vi "NACA_0015_Post_Proc.vi"(3 "Mode":T5, 5 "Traverse line In":T2 {"Row Duration (mins)" format="%#.1f"; "Row No" min=0; "Trace Gas Concentration (%)" min=0.0 format="%#.2f"; "Emission Rate (l/min)" format="%#.2f"; "Tunnel Speed" format="%#.2f"; "Start X" format="%#.2f"; "Start Y" format="%#.2f"; "Start Z" format="%#.2f"; "End X" format="%#.2f"; "End Y" format="%#.2f"; "End Z" format="%#.2f"; "Averaging time (min)" min=0.0 format="%#.2f"}) -> (0 "Error Message":string, 1 "Status":T1, 2 "Traverse line Out":T2 {"Row Duration (mins)" format="%#.1f"; "Row No" min=0; "Trace Gas Concentration (%)" min=0.0 format="%#.2f"; "Emission Rate (l/min)" format="%#.2f"; "Tunnel Speed" format="%#.2f"; "Start X" format="%#.2f"; "Start Y" format="%#.2f"; "Start Z" format="%#.2f"; "End X" format="%#.2f"; "End Y" format="%#.2f"; "End Z" format="%#.2f"; "Averaging time (min)" min=0.0 format="%#.2f"})   [LabVIEW 2011]
uses:
  Gen Trav/Traverse_cluster.ctl
  Gen Trav/Spacing.ctl
  Controls/Multi_run_mode.ctl
  Controls/User_Specific_mode.ctl
  Gen Trav/Multi_Run_Status.ctl
  Controls/File_Selector_Type.ctl
  <vilib>/Analysis/8numeric.llb/1D Numeric Integration.vi
  <vilib>/Analysis/NI_AALPro.lvlib
panel:
  out "Array":dbl[][](array[numeric])
  # "X           Y            Z"
  # "Start"
  # "End"
  # "X           Y            Z"
  # "Start"
  # "End"
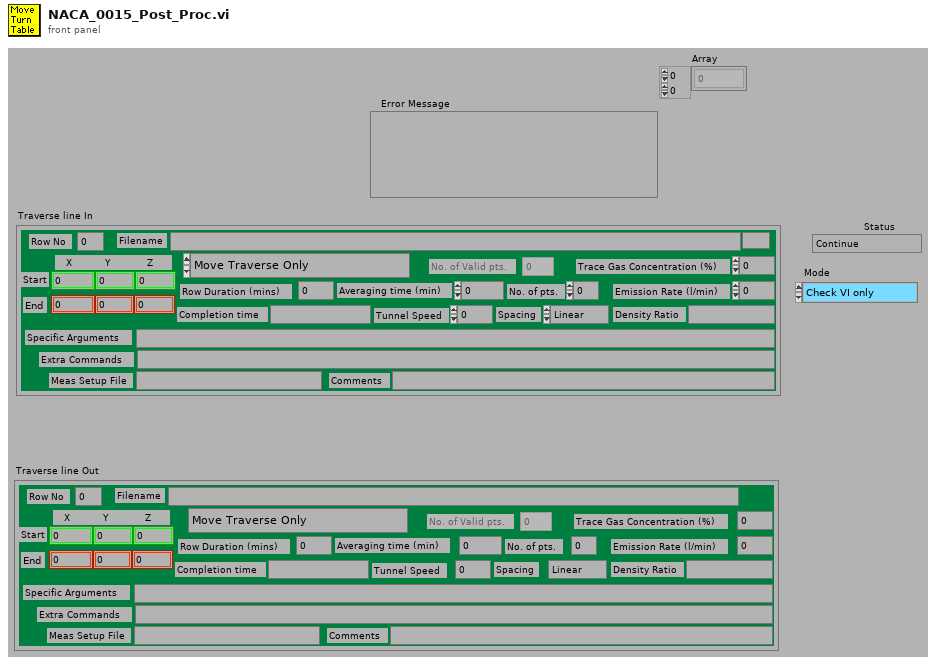
[diagram p1: front panel]
types:
  T1 = typedef "Multi_Run_Status.ctl" = enum16{"Continue", "Jump to Next Point", "Jump to Next Row", "Jump To Fall Back", "Terminate Run"}
  T2 = typedef "Traverse_cluster.ctl" = cluster{"Start X":dbl, "Start Y":dbl, "Start Z":dbl, "End X":dbl, "End Y":dbl, "End Z":dbl, "No. of pts.":i32, "Spacing":T3, "Filename":path, "Tunnel Speed":dbl, "Averaging time (min)":dbl, "Extra Commands":string, "Specific Arguments":string, "Emission Rate (l/min)":dbl, "Trace Gas Concentration (%)":dbl, "Density Ratio":string, "Comments":string, "Row No":i32, "Row Type Selector":T4, "Completion time":string, "Row Duration (mins)":dbl, "No. of Valid pts.":i32, "Meas Setup File":string}
  T3 = typedef "Spacing.ctl" = enum16{"Linear", "Log", "Gauss", "Specified", "N/A"}
  T4 = typedef "Multi_run_mode.ctl" = enum16{"Move Traverse Only", "Set Tunnel Speed Only", "Set Source Only", "Set Measurement Conditions", "Single Measurement", "Vertical Profile", "Lateral Profile", "Longitudinal Profile", "Explore Volume", "Multi-Axis Profile", "Auto Calibrate", "Meas Fast FID Bkgnd", "Check Beam Power", "Scanning Valve Measurement", "Run VI Named:", "Set ADAM Ch", "Wait (minutes)", "Send Message", "Synchronize With:", "Fall Back to this Row", "Turn Off Row Repeating", "Blank Row"}
  T5 = typedef "User_Specific_mode.ctl" = enum16{"Check VI only", "Run VI"}
  T6 = typedef "File_Selector_Type.ctl" = enum16{"The Selected File", "The Selected Folder", "Files containing the search string in the selected folder", "All files listed in selected file"}
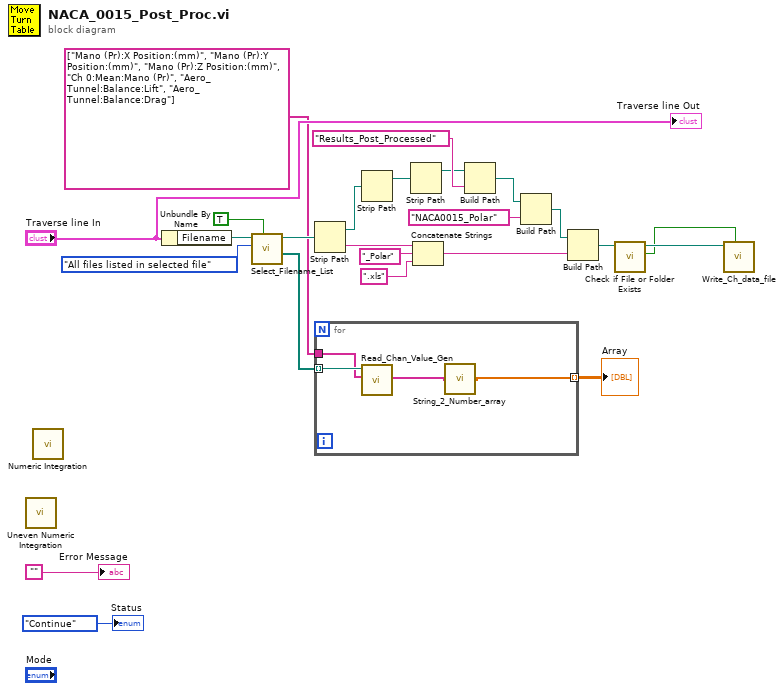
[diagram p0: block diagram]
diagram:
  n1 = call <vilib>:"Uneven Numeric Integration.vi"() -> ()  [unwired: 10 in, 2 out]
  n2 = call-poly <vilib>:"Numeric Integration.vi"() -> ()  [unwired: 3 in, 2 out]
  n3 = Unbundle By Name("Traverse line In") -> ("Filename"=w21:path)
  n4 = call "Select_Filename_List.vi"("No dialogs"=TRUE, "At Dialog Prompt Post Process"=File_Selector_Type."All files listed in selected file", "Previous Choice"=w21) -> ("Selected files"=w18:path[], "Choosen path"=w8:path)  [unwired: 3 in, 1 out]
  n5 = Strip Path(path=w8) -> (stripped path=w7:path, name=w6:string)
  n6 = for {
    tunnel: w18 -> [w28] mode=indexing
    tunnel: string[] ["Mano (Pr):X Position:(mm)", "Mano (Pr):Y Position:(mm)", "Mano (Pr):Z Position:(mm)", "Ch 0:Mean:Mano (Pr)", "Aero_Tunnel:Balance:Lift", "Aero_Tunnel:Balance:Drag"] -> [w27]
    tunnel: [w25] -> w1 mode=indexing
    n7 = call "Read_Chan_Value_Gen.vi"("Desired Ch Names"=w27, "Raw data file"=w28) -> ("Values"=w26:string[])  [unwired: 9 in]
    n8 = call "String_2_Number_array.vi"("Input String"=w26) -> ("Values"=w25:dbl[])
  }
  "Array" <- w1
  n9 = Strip Path(path=w7) -> (stripped path=w14:path)  [unwired: 1 out]
  n10 = Strip Path(path=w14) -> (stripped path=w15:path)  [unwired: 1 out]
  n11 = Concatenate Strings(w6, "_Polar" ("string"), ".xls" ("string")) -> (w17:string)
  n12 = Build Path(base path=w15, name or relative path="Results_Post_Processed") -> (appended path=w13:path)
  n13 = Build Path(base path=w13, name or relative path="NACA0015_Polar" ("New Results Folder Name")) -> (appended path=w12:path)
  n14 = Build Path(base path=w12, name or relative path=w17) -> (appended path=w10:path)
  n15 = call <vilib>:"Check if File or Folder Exists.vi"("path"=w10) -> ("file or folder exists?"=w5:bool, "dup path"=w9:path)  [unwired: 8 in, 1 out]
  n16 = call "Write_Ch_data_file.vi"("exists?"=w5, "Filename"=w9) -> ()  [unwired: 10 in]
  "Status" <- Multi_Run_Status."Continue" ("Status")
  "Traverse line Out" <- "Traverse line In"
  "Error Message" <- ""
